vi "Example - SLL CSV Logger.vi"() -> ()   [LabVIEW 2016, in "SLL Spreadsheet.lvlib" / "SLL CSV Logger.lvclass"]
doc: "Example for SLL CSV Logger with support for dynamically adding new headers/columns."
uses:
  SLL CSV Logger.lvclass
  _Typedefs/String Key Value Pair Cluster.ctl
  _Typedefs/Numeric Array Key Value Pair Cluster.ctl
  SLL Spreadsheet.lvlib
panel:
  in  "2D Data with Headers":string[][](array[string])=[["Header 2", "Header 6", "Header 7"], ["Data 2D - 2", "Data 2D - 6", "Data 2D - 7"]]
  in  "Numeric Array Key Value Pairs":T1[](array[typedef])=[{"Key"="Header 5", "Value"=[50.0, 51.0]}]
  out "2D Array Logged":string[][](array[string])
  in  "Key Value Pairs 2":T2[](array[typedef])=[{"Key"="Header 3", "Value"="KV 2 - 3"}, {"Key"="Header 2", "Value"="KV 2 - 2"}, {"Key"="Header 4", "Value"="KV 2 - 4"}]
  in  "Key Value Pairs 1":T2[](array[typedef])=[{"Key"="Header 1", "Value"="KV 1 - 1"}, {"Key"="Header 2", "Value"="KV 1 - 2"}]
  in  "Starter Headers[]":string[](array[string])=["Header 1", "Header 2", "Header 3"]
  in  "File Path":path=path "C:/Users/Public/Documents/SLL CSV Logger.csv"
  out "error out":errorcluster
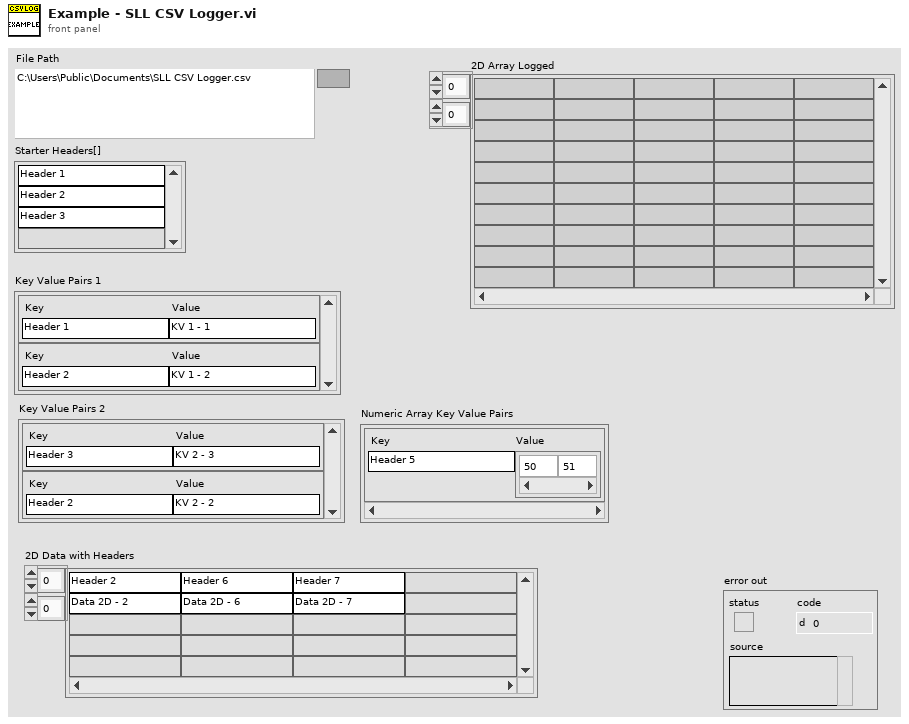
[diagram p1: front panel]
types:
  T1 = typedef "SLL Spreadsheet.lvlib/SLL CSV Logger.lvclass/Numeric Array Key Value Pair Cluster.ctl" = cluster{"Key":string, "Value":dbl[]}
  T2 = typedef "SLL Spreadsheet.lvlib/SLL CSV Logger.lvclass/String Key Value Pair Cluster.ctl" = cluster{"Key":string, "Value":string}
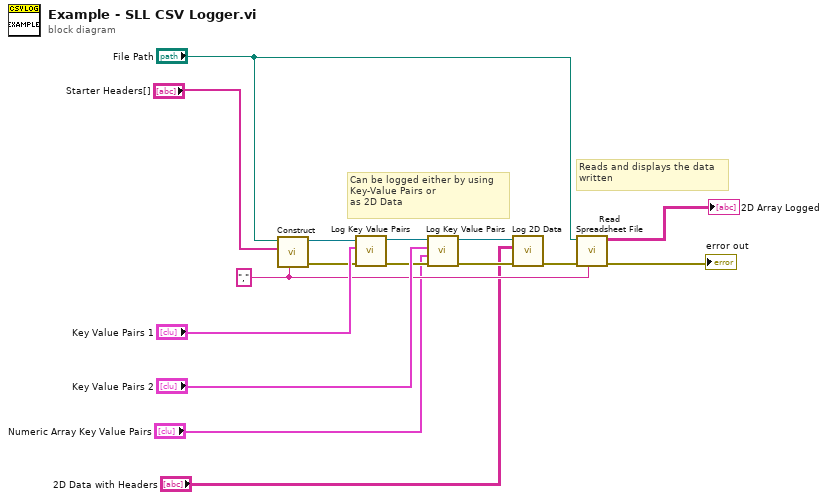
[diagram p0: block diagram]
diagram:
  w6 = "," ("Delimiter (,)")
  # "Reads and displays the data \nwritten"
  # "Can be logged either by using\nKey-Value Pairs or\nas 2D Data"
  n1 = call "Construct.vi"("Delimiter (,)"=w6, "Starter Headers[]"="Starter Headers[]", "File Path"="File Path") -> ("error out"=w12:errorcluster, "SLL CSV Logger out"=w11:refnum<class "SLL CSV Logger.lvclass">)  [unwired: 7 in]
  n2 = call "Log Key Value Pairs.vi"("error in (no error)"=w12, "String Key Value Pairs"="Key Value Pairs 1", "SLL Spreadsheet Logger in"=w11) -> ("error out"=w9:errorcluster, "SLL Spreadsheet Logger out"=w10:refnum<class "SLL CSV Logger.lvclass">)  [unwired: 7 in]
  n3 = call "Log Key Value Pairs.vi"("error in (no error)"=w9, "Numeric Array Key Value Pairs"="Numeric Array Key Value Pairs", "String Key Value Pairs"="Key Value Pairs 2", "SLL Spreadsheet Logger in"=w10) -> ("error out"=w16:errorcluster, "SLL Spreadsheet Logger out"=w2:refnum<class "SLL CSV Logger.lvclass">)  [unwired: 6 in]
  n4 = call "Log 2D Data.vi"("error in (no error)"=w16, "2D Data with Headers"="2D Data with Headers", "SLL Spreadsheet Logger in"=w2) -> ("error out"=w3:errorcluster)  [unwired: 7 in, 1 out]
  n5 = call "Read Spreadsheet File.vi"("Delimiter (tab)"=w6, "error in (no error)"=w3, "File Path"="File Path") -> ("error out"=→"error out":errorcluster, "2D Array"=→"2D Array Logged":string[][])  [unwired: 7 in]
